vi "Align Needle Dialog.vi"(7 "Console Log in":refnum<class "Console Log.lvclass">, 8 "error in":errorcluster, 11 "Potting Procedure in":refnum<class "Potting Procedure.lvclass">) -> (0 "error out":errorcluster, 2 "Canceled":bool, 3 "Potting Procedure out":refnum<class "Potting Procedure.lvclass">, 5 "Console Log out":refnum<class "Console Log.lvclass">)   [LabVIEW 2011]
uses:
  Procedure Classes/Potting Procedure/Potting Procedure.lvclass
  Application Utilities/Console Log/Console Log.lvclass
  Shared Components/Config Manager Class/Type Definitions/Named Position.ctl
  Shared Components/Gantry Class/Gantry Class.lvclass
  Shared Components/Config Manager Class/Type Definitions/Camera Enum.ctl
  Shared Components/Vec3d Class/Vec3d Class.lvclass
  Shared Components/Config Manager Class/Type Definitions/Offset.ctl
  Shared Components/WorkTable Class/WorkTable Class.lvclass
  Shared Components/Config Manager Class/Config Manager Class.lvclass
panel:
  out "Offset(mm)":cluster{"X":dbl, "Y":dbl, "Z":dbl}
  in  "Camera Selection":enum32{"Radio Selection 1", "Radio Selection 2"}(radio)
  out "preview":T1(plugin-control)
  in  "OK Button":bool
  in  "Cancel Button":bool
  # "Use the MPG  hand control to\nmove the needle tip to the center\nof the image in both X and Y"
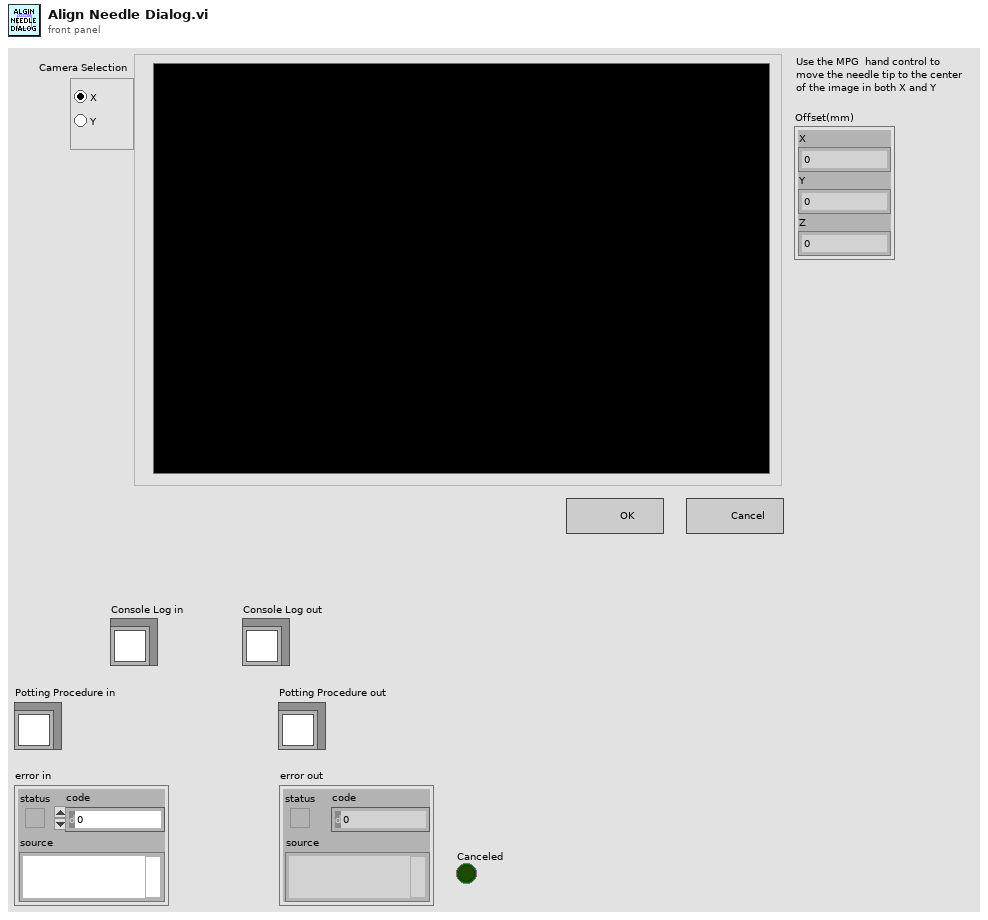
[diagram p1: front panel]
types:
  T1 = typedef "IMAQ Image.ctl" = refnum<image>
  T2 = typedef "Named Position.ctl" = enum16{"home", "module_chuck_0", "module_chuck_1", "module_chuck_2", "module_chuck_3", "module_chuck_4", "glue_reservoir_chuck", "stamp_tool_chuck", "weight_tool_chuck", "needle_calibration", "tool_rack_pos_0_in", "tool_rack_pos_0_out", "tool_rack_pos_1_in", "tool_rack_pos_1_out", "tool_rack_pos_2_in", "tool_rack_pos_2_out", "front_load_position", "grabber_start_pos", "between_chuck_0_and_1", "between_chuck_2_and_3"}
  T3 = enum8{"Enabled", "Disabled", "Disabled and Grayed Out"}
  T4 = typedef "Camera Enum.ctl" = enum16{"GANTRY HEAD", "NEEDLE CALIBRATION X", "NEEDLE CALIBRATION Y"}
  T5 = typedef "Physical Image.ctl" = cluster{"Image Position":refnum<class "Vec3d Class.lvclass">, "Image Reference":T1, "Field of View":cluster{"x(mm)":dbl, "y(mm)":dbl}}
  T6 = typedef "Offset.ctl" = enum16{"needle_offset", "tool_holder_offset"}
  T7 = typedef "Worktable_Syringe.ctl" = cluster{"Syringe Holder":enum16{"Empty", "Populated", "Calibrated"}, "Mixing Time":timestamp, "Tip Offset":refnum<class "Vec3d Class.lvclass">}
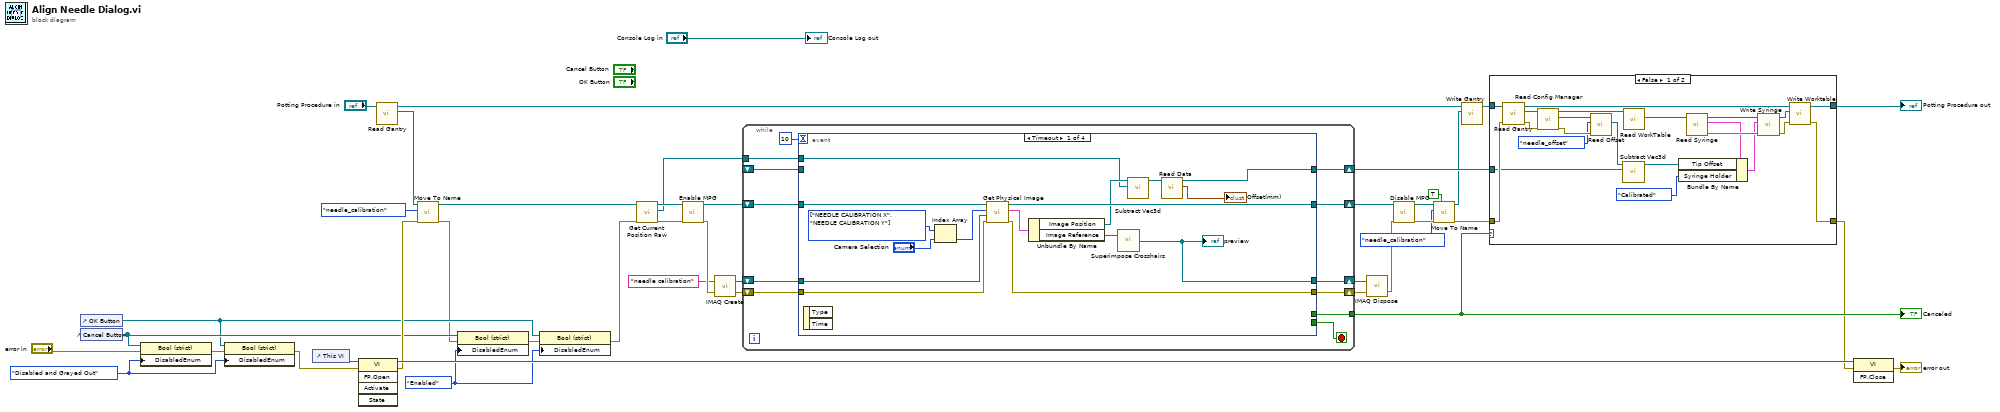
[diagram p0: block diagram]
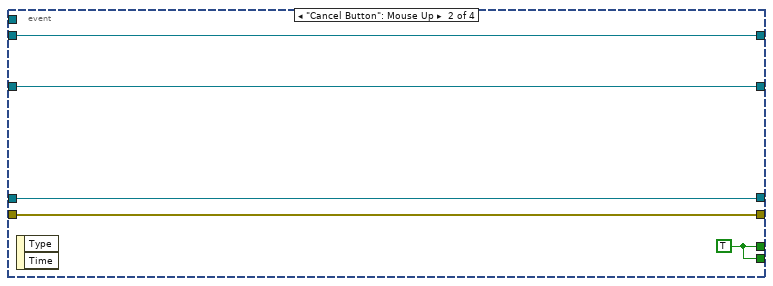
[diagram p3: hidden frame]
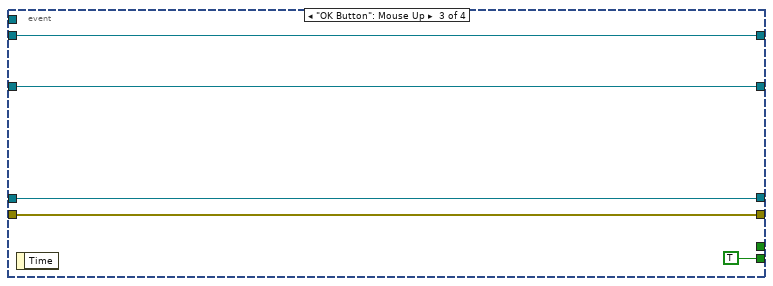
[diagram p4: hidden frame]
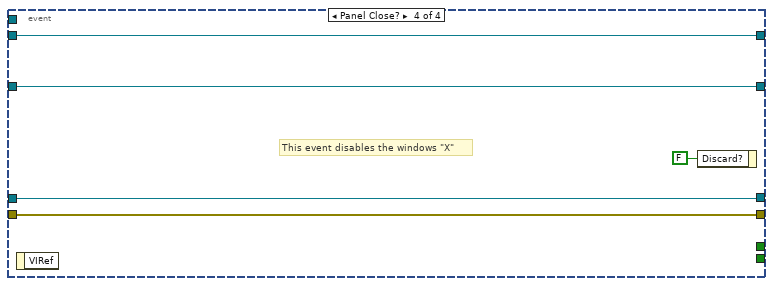
[diagram p5: hidden frame]
diagram:
  w8 = T3."Enabled" ("Disabled")
  w9 = T3."Disabled and Grayed Out" ("Disabled")
  n1 = control-ref of="OK Button"() -> (w10:refnum<vi>)
  n2 = control-ref of="Cancel Button"() -> (w11:refnum<vi>)
  n3 = property class="Bool (strict)"(reference=w11, error in="error in", "DisabledEnum"=w9) -> (error out=w13:errorcluster)  [unwired: 1 out]
  n4 = property class="Bool (strict)"(reference=w10, error in=w13, "DisabledEnum"=w9) -> (error out=w7:errorcluster)  [unwired: 1 out]
  n5 = control-ref of="This VI"() -> (w43:refnum<vi>)
  n6 = invoke class="VI" method="FP.Open"(reference=w43, error in=w7) -> (reference out=w42:refnum<vi>, error out=w38:errorcluster)  [unwired: 3 in, 3 out]
  n7 = call-dynamic "Read Gantry.vi"("Potting Procedure in"="Potting Procedure in") -> ("Gantry"=w39:refnum<class "Gantry Class.lvclass">, "Potting Procedure out"=w23:refnum<class "Potting Procedure.lvclass">)  [unwired: 8 in, 1 out]
  n8 = call-dynamic "Move To Name.vi"("error in"=w38, "Destination"=Named_Position."needle_calibration", "Gantry in"=w39) -> ("error out"=w5:errorcluster, "Gantry out"=w37:refnum<class "Gantry Class.lvclass">)  [unwired: 7 in]
  n9 = property class="Bool (strict)"(reference=w11, error in=w5, "DisabledEnum"=w8) -> (error out=w12:errorcluster)  [unwired: 1 out]
  n10 = property class="Bool (strict)"(reference=w10, error in=w12, "DisabledEnum"=w8) -> (error out=w4:errorcluster)  [unwired: 1 out]
  n11 = call-dynamic "Get Current Position Raw.vi"("error in"=w4, "Gantry in"=w37) -> ("error out"=w33:errorcluster, "Vec3d Class out"=w26:refnum<class "Vec3d Class.lvclass">, "Gantry out"=w36:refnum<class "Gantry Class.lvclass">)  [unwired: 7 in]
  n12 = call-dynamic "Enable MPG.vi"("error in"=w33, "Gantry in"=w36) -> ("error out"=w32:errorcluster, "Gantry out"=w35:refnum<class "Gantry Class.lvclass">)  [unwired: 8 in]
  n13 = call "IMAQ Create"("Image Name"="needle calibration", "error in (no error)"=w32) -> ("New Image"=w29:T1, "error out"=w30:errorcluster)  [unwired: 3 in]
  n14 = while {
    tunnel: [w51] -> w24
    shift-right: [w49] -> w34
    shift-left: w35 -> [w50]
    shift-right: [w53] -> w28
    shift-left: w30 -> [w52]
    shift-right: [w47] -> w27
    shift-left: w29 -> [w48]
    tunnel: w26 -> [w46]
    shift-right: [w45] -> w21
    shift-left: _ -> [w44]
    stop <- w54 stop-if-true
    n15 = event shown="[0] Timeout" {
      selector: _ -> [_ _ _ _]
      dyn-events: _ -> [_ _ _ _]
      timeout: 10 -> [_ _ _ _]
      tunnel: [_ w75 TRUE _] -> w54
      tunnel: [w62 w76 w81 w85] -> w53
      tunnel: w52 -> [w63 w76 w81 w85]
      tunnel: [_ w75 _ _] -> w51
      tunnel: w50 -> [w69 w73 w78 w83]
      tunnel: [w67 w73 w78 w83] -> w49
      tunnel: w48 -> [w64 w72 w77 w82]
      tunnel: [w61 w72 w77 w82] -> w47
      tunnel: w46 -> [w56 _ _ _]
      tunnel: [w58 w74 w79 w84] -> w45
      tunnel: w44 -> [_ w74 w79 w84]
      event Timeout {
        w70 = T4[] [enum."NEEDLE CALIBRATION X", enum."NEEDLE CALIBRATION Y"] items=["GANTRY HEAD", "NEEDLE CALIBRATION X", "NEEDLE CALIBRATION Y"]
        n16 = event-data() -> ()  [unwired: 1 in, 2 out]
        n17 = Index Array(array=w70, index="Camera Selection") -> (element=w68:T4)
        n18 = call-dynamic "Get Physical Image.vi"("error in"=w63, "Image In"=w64, "Camera Name"=w68, "Gantry in"=w69) -> ("error out"=w62:errorcluster, "Physical Image"=w66:T5, "Gantry out"=w67:refnum<class "Gantry Class.lvclass">)  [unwired: 5 in]
        n19 = Unbundle By Name(w66) -> ("Image Position"=w60:refnum<class "Vec3d Class.lvclass">, "Image Reference"=w65:T1)
        n20 = call "Superimpose Crosshairs.vi"("Refnum in"=w65) -> ("Refnum out"=w61:T1)  [unwired: 1 in]
        "preview" <- w61
        n21 = call "Subtract Vec3d.vi"("Vec3d in 2"=w56, "Vec3d in 1"=w60) -> ("Vec3d Class out"=w59:refnum<class "Vec3d Class.lvclass">)  [unwired: 8 in, 1 out]
        n22 = call-dynamic "Read Data.vi"("Vec3d Class in"=w59) -> ("Data"=→"Offset(mm)":cluster{"X":dbl, "Y":dbl, "Z":dbl}, "Vec3d Class out"=w58:refnum<class "Vec3d Class.lvclass">)  [unwired: 8 in, 1 out]
      }
      event "Cancel Button": Mouse Up {
        w75 = TRUE
        n23 = event-data() -> ()  [unwired: 1 in, 2 out]
      }
      event "OK Button": Mouse Up {
        n24 = event-data() -> ()  [unwired: 1 in, 1 out]
      }
      event Panel Close? {
        # "This event disables the windows \"X\""
        n25 = event-data() -> ()  [unwired: 1 in, 1 out]
        n26 = event-data("Discard?"=FALSE) -> ()  [unwired: 1 in, 1 out]
      }
    }
  }
  "Canceled" <- w24
  n27 = call "IMAQ Dispose"("Image"=w27, "error in (no error)"=w28) -> ("error out"=w25:errorcluster)  [unwired: 4 in]
  n28 = call-dynamic "Disable MPG.vi"("error in"=w25, "Gantry in"=w34) -> ("error out"=w18:errorcluster, "Gantry out"=w17:refnum<class "Gantry Class.lvclass">)  [unwired: 8 in]
  n29 = call-dynamic "Move To Name.vi"("Move if Same"=TRUE, "error in"=w18, "Destination"=Named_Position."needle_calibration", "Gantry in"=w17) -> ("error out"=w14:errorcluster, "Gantry out"=w15:refnum<class "Gantry Class.lvclass">)  [unwired: 6 in]
  n30 = call-dynamic "Write Gantry.vi"("Gantry"=w15, "Potting Procedure in"=w23) -> ("Potting Procedure out"=w22:refnum<class "Potting Procedure.lvclass">)  [unwired: 8 in, 1 out]
  n31 = case shown="False" w24 {
    tunnel: w14 -> [w102 w109]
    tunnel: w22 -> [w106 w110]
    tunnel: [w103 w110] -> w20
    tunnel: w21 -> [w101 _]
    tunnel: [w99 w109] -> w19
    frame False {
      n32 = call-dynamic "Read Gantry.vi"("error in (no error)"=w102, "Potting Procedure in"=w106) -> ("error out"=w92:errorcluster, "Gantry"=w94:refnum<class "Gantry Class.lvclass">, "Potting Procedure out"=w104:refnum<class "Potting Procedure.lvclass">)  [unwired: 7 in]
      n33 = call-dynamic "Read Config Manager.vi"("error in"=w92, "Gantry in"=w94) -> ("error out"=w95:errorcluster, "Config Manager"=w96:refnum<class "Config Manager Class.lvclass">, "Gantry out"=w93:refnum<class "Gantry Class.lvclass">)  [unwired: 7 in]
      n34 = call "Read Offset.vi"("error in"=w95, "Offset"=Offset."needle_offset", "Config Manager in"=w96) -> ("Vec3d out"=w89:refnum<class "Vec3d Class.lvclass">)  [unwired: 6 in, 2 out]
      n35 = call "Subtract Vec3d.vi"("Vec3d in 2"=w101, "Vec3d in 1"=w89) -> ("Vec3d Class out"=w97:refnum<class "Vec3d Class.lvclass">)  [unwired: 8 in, 1 out]
      n36 = call-dynamic "Read WorkTable.vi"("Gantry Class in"=w93) -> ("WorkTable Class.lvclass"=w91:refnum<class "WorkTable Class.lvclass">)  [unwired: 8 in, 2 out]
      n37 = call "Read Syringe.vi"("WorkTable in"=w91) -> ("error out"=w107:errorcluster, "Syringe"=w88:T7, "WorkTable out"=w108:refnum<class "WorkTable Class.lvclass">)  [unwired: 8 in]
      n38 = Bundle By Name(cluster=w88, "Tip Offset"=w97, "Syringe Holder"=enum16{"Empty", "Populated", "Calibrated"}."Calibrated") -> (w87:T7)
      n39 = call-dynamic "Write Syringe.vi"("error in (no error)"=w107, "Syringe"=w87, "WorkTable Class in"=w108) -> ("error out"=w100:errorcluster, "WorkTable Class out"=w105:refnum<class "WorkTable Class.lvclass">)  [unwired: 7 in]
      n40 = call-dynamic "Write Worktable.vi"("error in"=w100, "WorkTable in"=w105, "Potting Procedure in"=w104) -> ("error out"=w99:errorcluster, "Potting Procedure out"=w103:refnum<class "Potting Procedure.lvclass">)  [unwired: 7 in]
    }
    frame True {
    }
  }
  "Potting Procedure out" <- w20
  n41 = invoke class="VI" method="FP.Close"(reference=w42, error in=w19) -> (error out=→"error out":errorcluster)  [unwired: 1 in, 2 out]
  "Console Log out" <- "Console Log in"
